vi "RT Loop - Acquire camera_data_2.vi"(8 "Boolean":bool, 11 "Message Queue":refnum<queue>) -> ()   [LabVIEW 2017]
uses:
  UI Error Handlers/support/Message Queue/Message Cluster.ctl
  <vilib>/vision/Image Controls.llb/IMAQ Image.ctl
  <vilib>/userdefined/High Color/IMAQdx.ctl
  <vilib>/vision/Avi.llb/IMAQ AVI2 Codec Path.ctl
  Globals/Global - All RT Loop Stop.vi
  Globals/Global - Configuration Options.vi
  <vilib>/vision/driver/NI_Vision_Acquisition_Software.lvlib
  UI Error Handlers/support/Message Queue/Message Queue.lvlib
panel:
  out "Webcam":T1(plugin-control)
  out "Cluster":cluster{"Image Out":T1, "AVI Path 2":path}
  out "AVI Path":path
  out "Acceleration Log Folder":path=path "/home/lvuser/Log/logfiles_deploy"
  out "Codec Names":string[](array[string])
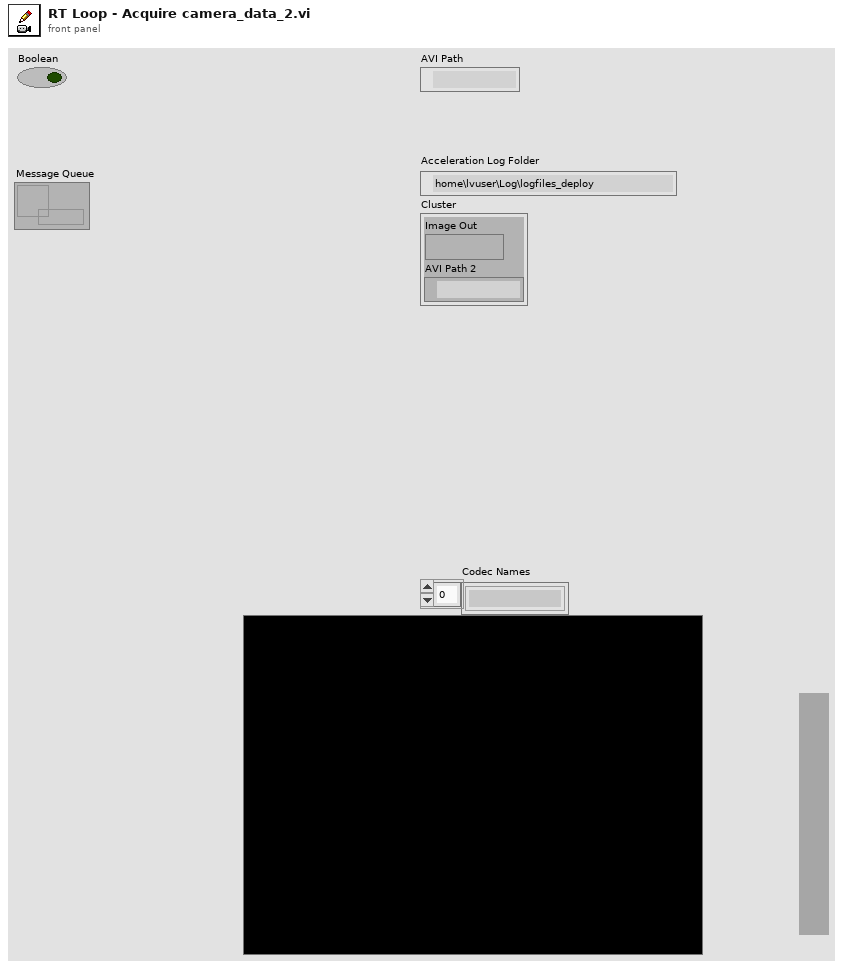
[diagram p1: front panel]
types:
  T1 = typedef "IMAQ Image.ctl" = refnum<image>
  T2 = typedef "IMAQdx.ctl" = refnum<k21>
  T3 = typedef "Image Type" = u32
  T4 = typedef "IMAQ AVI2 Codec Path.ctl" = u32
  T5 = cluster{"Tool data":cluster{"Number of teeth":sgl}, "Cutting data":cluster{"rpm":sgl}, "Limits":cluster{"Magnitude threshold":sgl, "Tolerance":sgl}, "G1 status":cluster{"G1 trigger":bool}}
  T6 = typedef "IMAQ AVI2 Refnum.ctl" = refnum<k20>
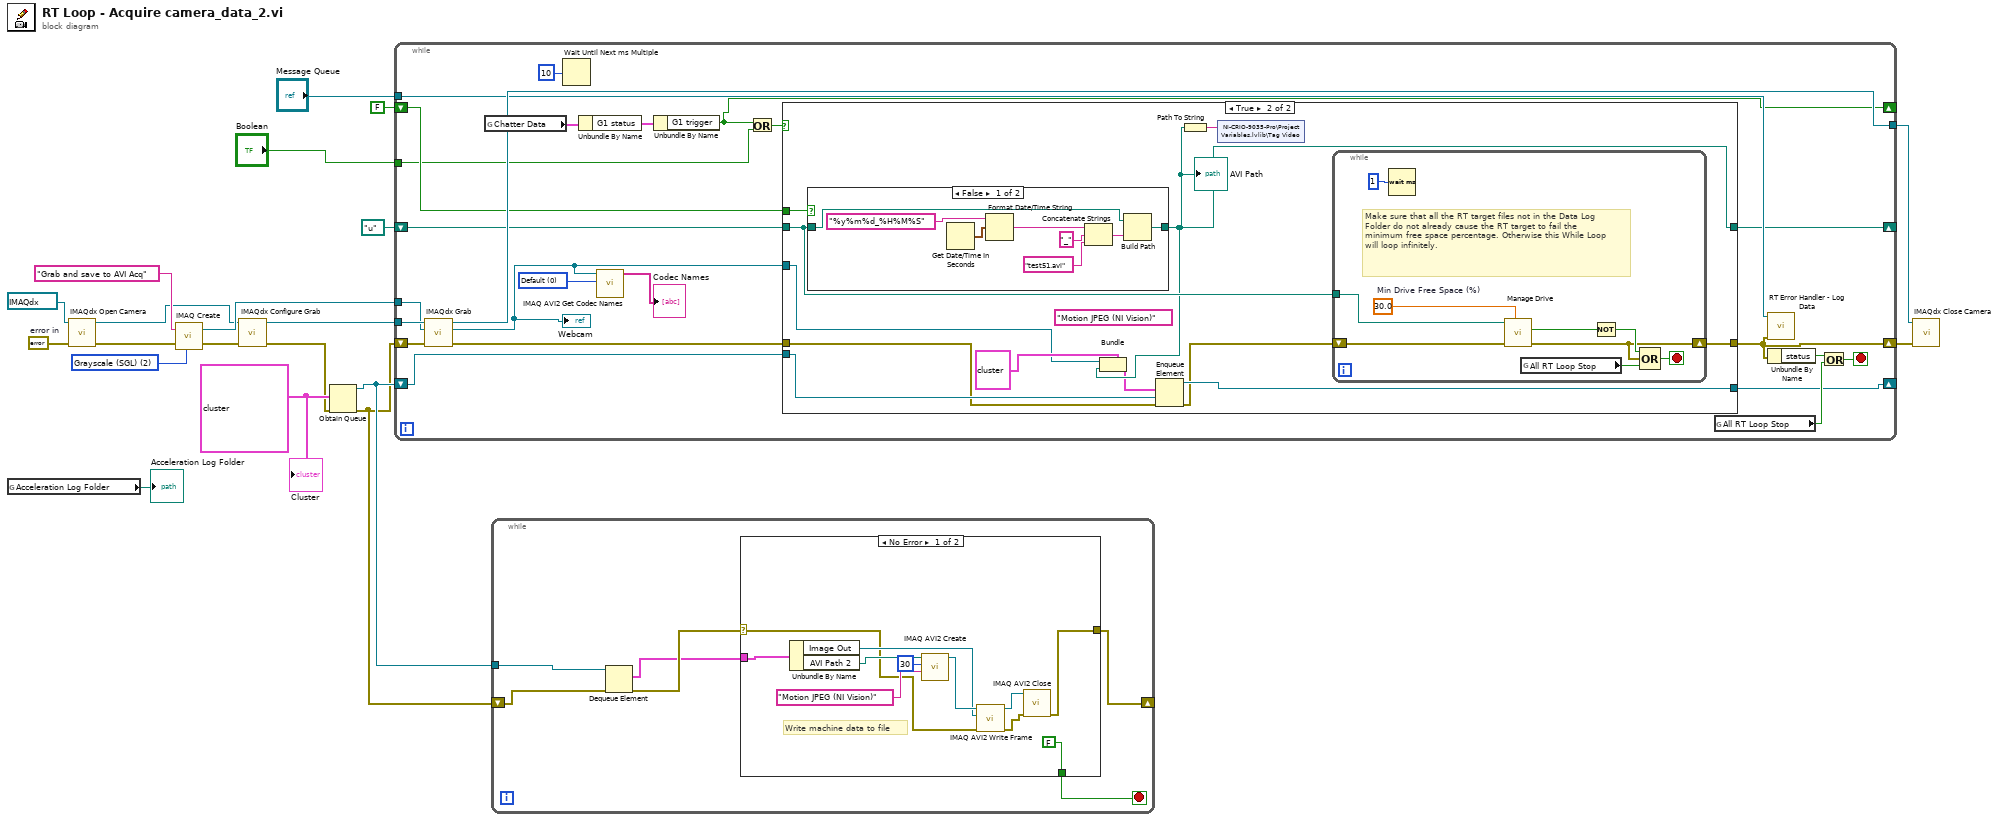
[diagram p0: block diagram]
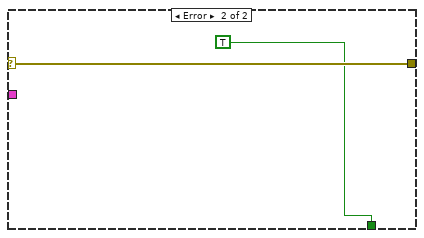
[diagram p2: hidden frame]
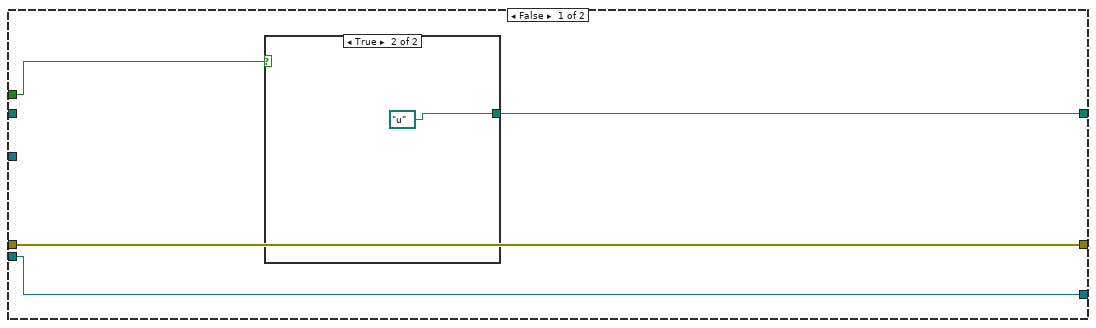
[diagram p3: hidden frame]
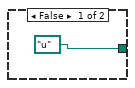
[diagram p4: hidden frame]
diagram:
  w4 = cluster{"Image Out":T1, "AVI Path 2":path} {"Image Out"=refnum, "AVI Path 2"=path ""}
  w17 = T3 2 items=["Grayscale (U8)", "Grayscale (I16)", "Grayscale (SGL)", "Complex (CSG)", "RGB (U32)", "HSL (U32)", "RGB (U64)", "Grayscale (U16)"] ("Image Type")
  w15 = errorcluster {"status"=FALSE, "code"=0, "source"=""}  # error in
  n1 = global read "Global - Configuration Options.vi" "Acceleration Log Folder"() -> (→"Acceleration Log Folder":path)
  n2 = call <vilib>:"IMAQdx Open Camera.vi"("error in"=w15, "Session In"=T2 "cam0") -> ("error out"=w18:errorcluster, "Session Out"=w13:T2)  [unwired: 8 in]
  n3 = call "IMAQ Create"("Image Name"="Grab and save to AVI Acq", "Image Type"=w17, "error in (no error)"=w18) -> ("New Image"=w20:T1, "error out"=w7:errorcluster)  [unwired: 2 in]
  n4 = call <vilib>:"IMAQdx Configure Grab.vi"("error in"=w7, "Session In"=w13) -> ("error out"=w3:errorcluster, "Session Out"=w19:T2)  [unwired: 8 in]
  n5 = Obtain Queue(element data type=w4, error in (no error)=w3) -> (queue out=w5:refnum<queue>, error out=w2:errorcluster)  [unwired: 3 in, 1 out]
  n6 = while {
    tunnel: w19 -> [w43]
    tunnel: w20 -> [w42]
    tunnel: [w41] -> w12
    tunnel: "Message Queue" -> [w33]
    shift-right: [w24] -> _
    shift-left: FALSE ("G1 trigger") -> [w29]
    shift-right: [w28] -> _
    shift-left: path "u:/" ("AVI Path") -> [w35]
    tunnel: "Boolean" -> [w27]
    shift-right: [w25] -> _
    shift-left: w5 -> [w26]
    shift-right: [w23] -> w1
    shift-left: w2 -> [w44]
    stop <- w39 stop-if-true
    w38 = T4 0 items=["Default", "System", "Built in Vision"] ("Codec Source")
    n7 = call <vilib>:"IMAQdx Grab.vi"("error in"=w44, "Image In"=w42, "Session In"=w43) -> ("error out"=w36:errorcluster, "Image Out"=w21:T1, "Session Out"=w41:T2)  [unwired: 5 in, 1 out]
    "Webcam" <- w21
    n8 = global read "Global - Configuration Options.vi" "Chatter Data"() -> (w32:T5)
    n9 = Wait Until Next ms Multiple(millisecond multiple=u32 10) -> ()  [unwired: 1 out]
    n10 = Unbundle By Name(w32) -> ("G1 status"=w31:cluster{"G1 trigger":bool})
    n11 = call "IMAQ AVI2 Get Codec Names"("Codec Source"=w38, "Image"=w21) -> ("Codec Names"=→"Codec Names":string[])  [unwired: 8 in, 1 out]
    n12 = Unbundle By Name(w31) -> ("G1 trigger"=w24:bool)
    n13 = Or(x=w24, y=w27) -> (x .or. y?=w30:bool)
    n14 = case shown="True" w30 {
      tunnel: w21 -> [_ w55]
      tunnel: w36 -> [w48 w51]
      tunnel: [w48 w62] -> w23
      tunnel: w35 -> [_ w61]
      tunnel: w29 -> [w47 w60]
      tunnel: [w46 w54] -> w28
      tunnel: w26 -> [w45 w58]
      tunnel: [w45 w57] -> w25
      frame False {
        n15 = case shown="True" w47 {
          tunnel: [path "u:/" ("AVI Path") path "u:/" ("AVI Path")] -> w46
          frame False {
          }
          frame True {
          }
        }
      }
      frame True {
        (unwired) "Motion JPEG (NI Vision)" ("Codec")
        n16 = case shown="False" w60 {
          tunnel: w61 -> [w64 w71]
          tunnel: [w63 w71] -> w54
          frame False {
            n17 = Get Date/Time In Seconds() -> (seconds since 1Jan1904=w66:timestamp)
            n18 = Format Date/Time String(time format string (%c)="%y%m%d_%H%M%S", seconds (now)=w66) -> (date/time string=w67:string)  [unwired: 1 out]
            n19 = Concatenate Strings(w67, "_" ("string"), "test51.avi" ("name or relative path")) -> (w70:string)
            n20 = Build Path(base path=w64, name or relative path=w70) -> (appended path=w63:path)
          }
          frame True {
          }
        }
        "AVI Path" <- w54
        n21 = Bundle(cluster=cluster{"Image Out":T1, "AVI Path 2":path} {"Image Out"=refnum, "AVI Path 2"=path ""} ("Cluster 2"), "Image Out"=w55, "AVI Path 2"=w54) -> (w53:cluster{"Image Out":T1, "AVI Path 2":path})
        n22 = Enqueue Element(queue=w58, element=w53, error in (no error)=w51) -> (queue out=w57:refnum<queue>, error out=w52:errorcluster)  [unwired: 1 in, 1 out]
        n23 = Path To String(path=w54) -> (string=w59:string)
        n24 = shared-variable "NI-CRIO-9035-Pro\\Project Variables.lvlib\\Tag Video"(w59) -> ()  [unwired: 1 in, 1 out]
        n25 = while {
          shift-right: [w75] -> w62
          shift-left: w52 -> [w76]
          tunnel: w61 -> [w73]
          stop <- w80 stop-if-true
          w74 = 30.0  # Min Drive Free Space (%)
          # "Make sure that all the RT target files not in the Data Log Folder do not already cause the RT target to fail the minimum free space percentage. Otherwise this While Loop will loop infinitely."
          n26 = Wait (ms)(milliseconds to wait=u32 1) -> ()  [unwired: 1 out]
          n27 = call "Manage Drive.vi"("Min Drive Free Space (%)"=w74, "error in"=w76, "Data Folder"=w73) -> ("error out"=w75:errorcluster, "Drive Space Below Limit"=w72:bool)  [unwired: 7 in]
          n28 = global read "Global - All RT Loop Stop.vi" "All RT Loop Stop"() -> (w77:bool)
          n29 = Not(x=w72) -> (.not. x?=w79:bool)
          n30 = Compound Arithmetic op=OR(w79, w75, w77) -> (w80:bool)
        }
      }
    }
    n31 = global read "Global - All RT Loop Stop.vi" "All RT Loop Stop"() -> (w34:bool)
    n32 = call "RT Error Handler - Log Data.vi"("error in (no error)"=w23, "Message Queue"=w33) -> ()  [unwired: 9 in, 1 out]
    n33 = Unbundle By Name(w23) -> ("status"=w40:bool)
    n34 = Or(x=w40, y=w34) -> (x .or. y?=w39:bool)
  }
  n35 = while {
    tunnel: w5 -> [w86]
    shift-right: [w82] -> _
    shift-left: w2 -> [w83]
    stop <- w81 stop-if-true
    n36 = Dequeue Element(queue=w86, error in (no error)=w83) -> (element=w84:cluster{"Image Out":T1, "AVI Path 2":path}, error out=w85:errorcluster)  [unwired: 1 in, 2 out]
    n37 = case shown="No Error" w85 {
      selector: w85 -> [w91 w99]
      tunnel: [w87 w99] -> w82
      tunnel: w84 -> [w97 _]
      tunnel: [FALSE TRUE] -> w81
      frame No Error {
        # "Write machine data to file"
        n38 = Unbundle By Name(w97) -> ("Image Out"=w92:T1, "AVI Path 2"=w96:path)
        n39 = call "IMAQ AVI2 Create"("Codec"="Motion JPEG (NI Vision)", "Frames Per Second"=u32 30, "AVI Path"=w96) -> ("AVI Refnum"=w93:T6)  [unwired: 7 in, 1 out]
        n40 = call "IMAQ AVI2 Write Frame"("error in (no error)"=w91, "Image"=w92, "AVI Refnum"=w93) -> ("error out"=w88:errorcluster, "AVI Refnum (duplicate)"=w89:T6)  [unwired: 6 in, 1 out]
        n41 = call "IMAQ AVI2 Close"("error in (no error)"=w88, "AVI Refnum"=w89) -> ("error out"=w87:errorcluster)  [unwired: 9 in]
      }
      frame Error {
      }
    }
  }
  n42 = call <vilib>:"IMAQdx Close Camera.vi"("error in"=w1, "Session In"=w12) -> ()  [unwired: 9 in, 1 out]
  "Cluster" <- w4
